vi "Set Full Image.vi"(10 "vbin":i32, 11 "hbin":i32) -> (3 "function return":u32)   [LabVIEW 2018, in "AndorSDK.lvlib"]
doc: "EXPNETTYPE unsigned int WINAPI SetFullImage(int hbin, int vbin);"
uses:
  AndorSDK.lvlib
  ATMCD32D.dll
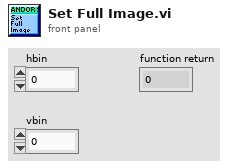
[diagram p1: front panel]
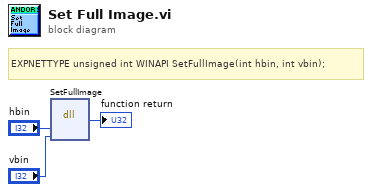
[diagram p0: block diagram]
diagram:
  # "EXPNETTYPE unsigned int WINAPI SetFullImage(int hbin, int vbin);"
  n1 = dll-call lib="PTH2babs E\nPersönliches02 - Arbeit03-HiwijobsLabviewCodelibANDOR\tAndor SDK\nATMCD32D.*" fn="SetFullImage"("hbin"="hbin", "vbin"="vbin") -> (→"function return":u32)  [unwired: 5 in, 2 out]
